vi "PQprint.vi"(8 "error in (no error)":errorcluster, 9 "ps":T1, 10 "res":u32, 11 "Refnum (Eingang)":refnum<file>) -> (0 "error out":errorcluster, 3 "Refnum (Ausgang)":refnum<file>)   [LabVIEW 2019, in "libpqlv.lvlib"]
uses:
  libpqlv.lvlib
  libpq.dll
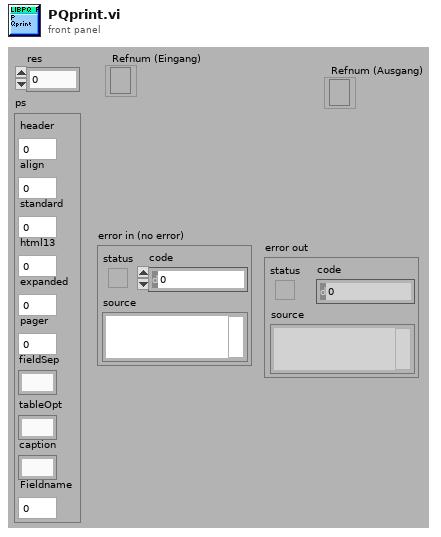
[diagram p1: front panel]
types:
  T1 = cluster{"fieldSep":string, "tableOpt":string, "caption":string, "header":dbl, "align":dbl, "standard":dbl, "html13":dbl, "expanded":dbl, "pager":dbl, "Fieldname":dbl}
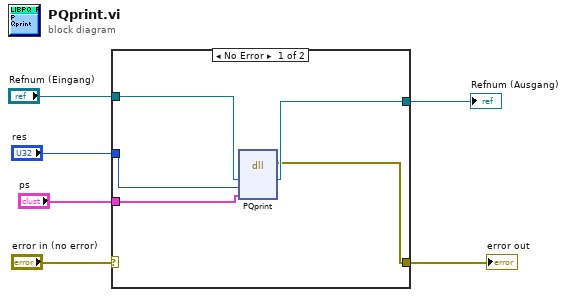
[diagram p0: block diagram]
diagram:
  n1 = case shown="No Error" "error in (no error)" {
    selector: "error in (no error)" -> [_ w13]
    tunnel: [w8 w13] -> w5
    tunnel: "res" -> [w11 _]
    tunnel: "Refnum (Eingang)" -> [w10 w12]
    tunnel: [w9 w12] -> w2
    tunnel: "ps" -> [w7 _]
    frame No Error {
      n2 = dll-call lib="libpq.*" fn="PQprint"("fout"=w10, "res"=w11, "ps"=w7) -> (error out=w8:errorcluster, "fout"=w9:refnum<file>)  [unwired: 6 in, 1 out]
    }
    frame Error {
    }
  }
  "error out" <- w5
  "Refnum (Ausgang)" <- w2
